vi "Write Directory Path.vi"(8 "error in (no error)":errorcluster, 10 "Directory Path":path, 11 "MeasurementSMO in":refnum<class "AFM_Litho_Plugin.IV.lvclass">) -> (0 "error out":errorcluster, 3 "MeasurementSMO out":refnum<class "AFM_Litho_Plugin.IV.lvclass">)   [LabVIEW 2019, in "AFM_Litho_Plugin.IV.lvclass"]
uses:
  AFM_Litho_Plugin.IV.lvclass
  AFM_Litho_Plugin.IV.lvclass/AFM_Litho_Plugin.IV.ctl
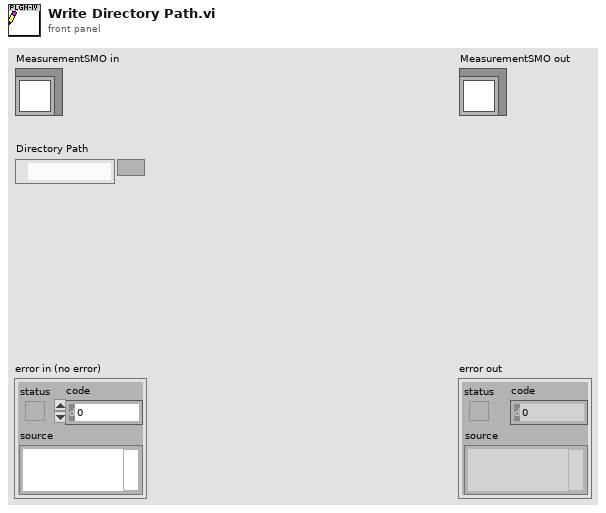
[diagram p1: front panel]
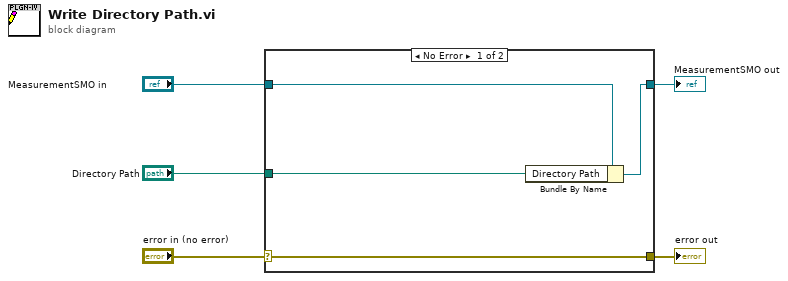
[diagram p0: block diagram]
diagram:
  n1 = case shown="No Error" "error in (no error)" {
    selector: "error in (no error)" -> [w9 w10]
    tunnel: [w9 w10] -> w4
    tunnel: [w7 w11] -> w2
    tunnel: "MeasurementSMO in" -> [w8 w11]
    tunnel: "Directory Path" -> [w6 _]
    frame No Error {
      n2 = Bundle By Name(cluster=w8, "Directory Path"=w6) -> (w7:refnum<class "AFM_Litho_Plugin.IV.lvclass">)
    }
    frame Error {
    }
  }
  "error out" <- w4
  "MeasurementSMO out" <- w2
